vi "Przełącznik J-K.vi"(6 "R":bool, 9 "K":bool, 10 "C":bool, 11 "J":bool) -> (2 "~Q":bool, 3 "Q":bool)   [LabVIEW 2020]
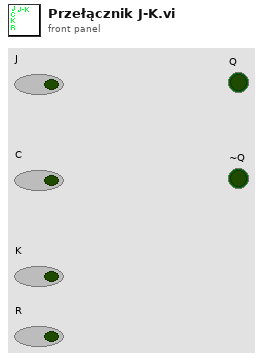
[diagram p1: front panel]
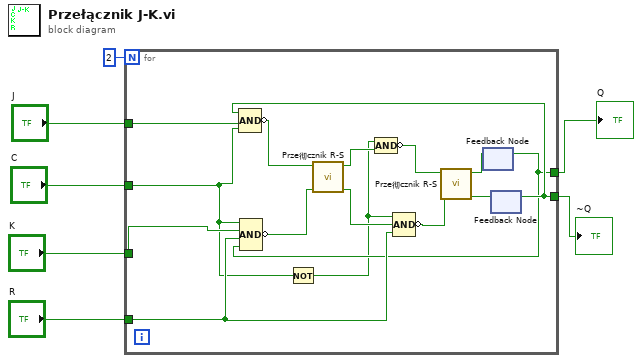
[diagram p0: block diagram]
diagram:
  n1 = for {
    N: 2 -> [_]
    tunnel: "J" -> [w21]
    tunnel: "C" -> [w8]
    tunnel: "K" -> [w20]
    tunnel: "R" -> [w19]
    tunnel: [w10] -> w6
    tunnel: [w12] -> w7
    n2 = Not(x=w8) -> (.not. x?=w9:bool)
    n3 = feedback #1() -> (w10:bool)  [unwired: 1 in]
    n4 = Compound Arithmetic op=AND(w8, w20, w19, w10) -> (invert w18:bool)
    n5 = feedback #2() -> (w12:bool)  [unwired: 1 in]
    n6 = Compound Arithmetic op=AND(w12, w21, w8) -> (invert w22:bool)
    n7 = call "Prze彻cznik R-S.vi"("S"=w18, "R"=w22) -> ("~Q"=w14:bool, "Q"=w17:bool)  [unwired: 8 in]
    n8 = Compound Arithmetic op=AND(w9, w17) -> (invert w16:bool)
    n9 = Compound Arithmetic op=AND(w9, w14, w19) -> (invert w15:bool)
    n10 = call "Prze彻cznik R-S.vi"("S"=w15, "R"=w16) -> ("~Q"=w13:bool, "Q"=w11:bool)  [unwired: 8 in]
    n11 = feedback-in #1(w11) -> ()
    n12 = feedback-in #2(w13) -> ()
  }
  "Q" <- w6
  "~Q" <- w7
